vi "AudioStreamer.Globals.vi"() -> ()   [LabVIEW 2020]
uses:
  AudioStreamer.Config.ctl
panel:
  in  "config":T1
  out "trig":bool
  out "running":bool
  out "last error":errorcluster
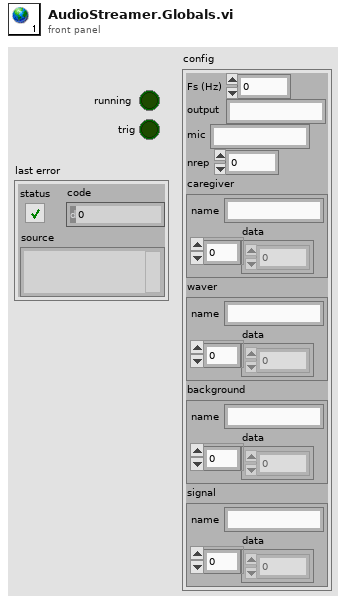
[diagram p1: front panel]
types:
  T1 = typedef "AudioStreamer.Config.ctl" = cluster{"Fs (Hz)":dbl, "output":string, "mic":string, "nrep":i32, "caregiver":cluster{"name":string, "data":sgl[]}, "waver":cluster{"name":string, "data":sgl[]}, "background":cluster{"name":string, "data":sgl[]}, "signal":cluster{"name":string, "data":sgl[]}}
diagram:
